vi "Concat string array.vi"(10 "String Array In":string[](array[string])) -> (2 "Concat Array Out":string[](array[string]))   [LabVIEW 2024, in "LVarex.lvlib"]
uses:
  LVarex.lvlib
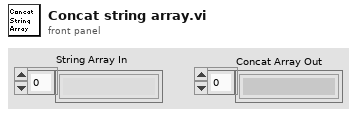
[diagram p1: front panel]
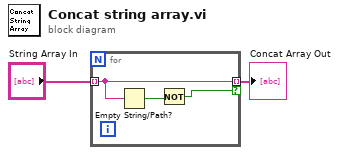
[diagram p0: block diagram]
diagram:
  n1 = for {
    tunnel: "String Array In" -> [w5] mode=indexing
    tunnel: [w5] -> w1 mode=indexing if=w3
    n2 = Empty String/Path?(string/path=w5) -> (empty?=w4:bool)
    n3 = Not(x=w4) -> (.not. x?=w3:bool)
  }
  "Concat Array Out" <- w1
